vi "Configure Measurement.vi"(6 "rate (0:slow)":u16(ring) items=["slow", "medium", "fast"], 8 "error in (no error)":errorcluster, 9 "range (0:auto)":u16(ring) items=["autorange", "200mV, 200 ohms", "2V, 2 kohms", "20V, 20 kohms", "200V, 200 kohms", "1000Vdc, 700 Vac, 2 Mohms", "20 Mohms", "20 mV, 20 ohms"], 10 "function (0:volts DC)":u16(ring) items=["volts DC", "volts AC", "2-wire k.ohms", "4-wire k.ohms", "mA DC", "mA AC"], 11 "VISA resource name":refnum<visa-resource-name>) -> (0 "error out":errorcluster, 3 "VISA resource name out":refnum<visa-resource-name>)   [LabVIEW 2009, in "Fluke 8840.lvlib"]
doc: "This VI configures the function, range and reading rate of the Fluke 8842A digital multimeter. This configuration VI works on the 8840A as well. The only difference in the two configure VIs is that the FL8842A Configure has one more optional range setting than the FL8840A. Therefore, the range setting \"20mV, 20 ohms\" will not work on the 8840A."
uses:
  Fluke 8840.lvlib
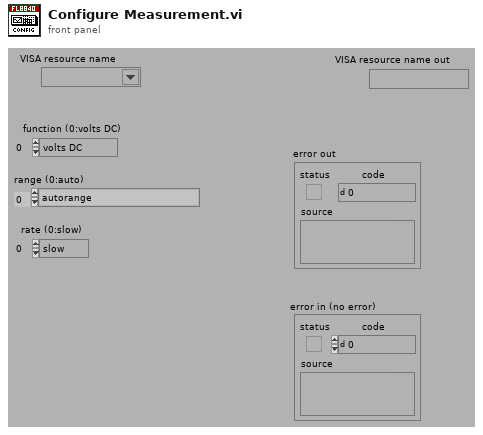
[diagram p1: front panel]
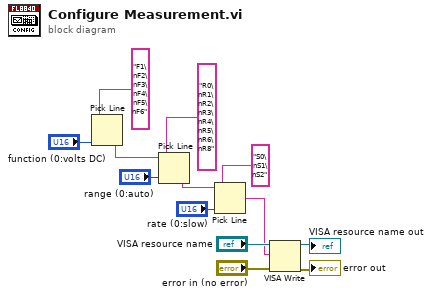
[diagram p0: block diagram]
diagram:
  n1 = Pick Line(multi-line string="F1\nF2\nF3\nF4\nF5\nF6", line index="function (0:volts DC)") -> (output string=w8:string)  [unwired: 1 out]
  n2 = Pick Line(string ("")=w8, multi-line string="R0\nR1\nR2\nR3\nR4\nR5\nR6\nR8", line index="range (0:auto)") -> (output string=w5:string)
  n3 = Pick Line(string ("")=w5, multi-line string="S0\nS1\nS2", line index="rate (0:slow)") -> (output string=w1:string)
  n4 = VISA Write(VISA resource name="VISA resource name", write buffer=w1, error in (no error)="error in (no error)") -> (VISA resource name out=→"VISA resource name out":refnum<visa-resource-name>, error out=→"error out":errorcluster)  [unwired: 1 out]
